vi "Word Report.vi"(6 "מק\"ט המכלל":string, 7 "עבר/נכשל":string="עבר/נכשל", 8 "מספר סידורי":string, 9 "שם הצב\"ד":string="שם הצב\"ד", 10 "מפעיל":string="ANS", 11 "Array":string[][](array[string])=[["Content", "Results", "Range", "Pass/Fail", "11"], ["Content", "Results", "Range", "Pass/Fail", "22"], ["Content", "Results", "Range", "Pass/Fail", "33"], ["Content", "Results", "Range", "Pass/Fail", "44"], ["Content", "Results", "Range", "Pass/Fail", "55"], ["55", "Content", "Results", "Range", "Pass/Fail"]]) -> ()   [LabVIEW 2014]
uses:
  <vilib>/addons/_office/_exclsub.llb/font.ctl
  <vilib>/addons/_office/word.llb/Word Easy Table (str).vi
  <vilib>/addons/_office/word.llb/Word Edit Cell ([str]).vi
  <vilib>/addons/_office/NI_ReportGenerationToolkit.lvlib
  <vilib>/Utility/NIReport.llb/Word/NI_Word.lvclass
panel:
  in  "start (0, 0)":cluster{"row":i32, "column":i32}={"row"=1, "column"=4}
  in  "value 3":string[][](array[string])
  in  "new element/subarray 3":string[](array[string])
  in  "new element/subarray":string[](array[string])
  in  "value":string[][](array[string])
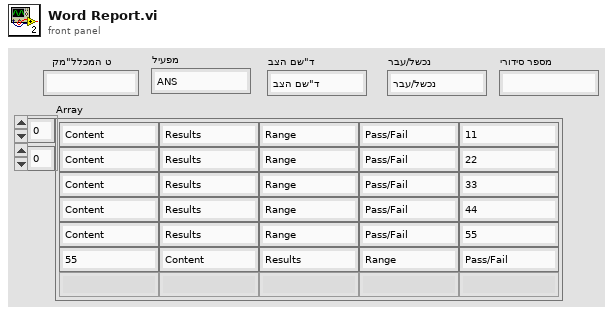
[diagram p1: front panel]
types:
  T1 = typedef "NI_ReportGenerationToolkit.lvlib/font.ctl" = cluster{"font name":string, "font size":dbl, "bold":u16, "italic":u16, "underline":u16, "strike through":u16, "font color":u32}
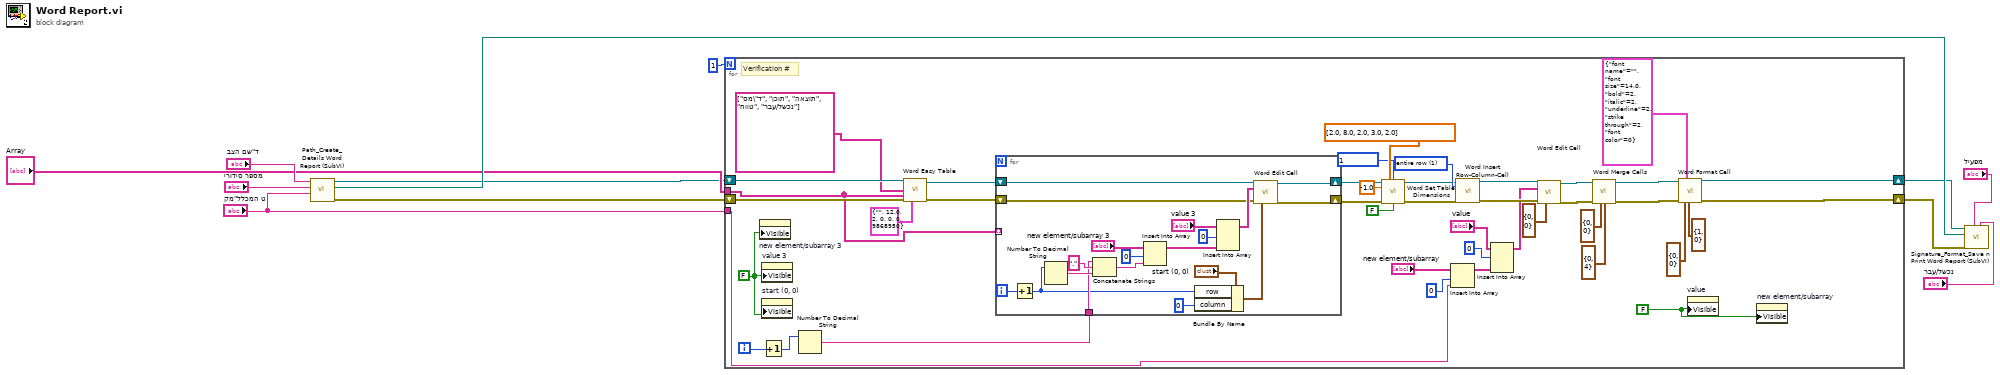
[diagram p0: block diagram]
diagram:
  n1 = call "Path_Create_Details Word Report (SubVI).vi"("שם ומק\"ט המכלל"="מק\"ט המכלל", "מספר סידורי"="מספר סידורי", "שם הצב\"ד"="שם הצב\"ד") -> ("error out"=w4:errorcluster, "Path"=w11:path, "NI_report out"=w5:refnum<class "NI_report.lvclass">)  [unwired: 6 in]
  n2 = for {
    N: 1 -> [_]
    shift-right: [w22] -> w9
    shift-left: w4 -> [w54]
    shift-right: [w23] -> w10
    shift-left: w5 -> [w53]
    tunnel: "Array" -> [w26]
    tunnel: "מק\"ט המכלל" -> [w14]
    i -> [w33]
    w34 = FALSE
    w40 = FALSE
    w52 = u16 1 items=["shift cells right", "entire row", "entire column"] ("mode (entire column)")
    # "Verification #"
    n3 = property on="new element/subarray 3" class="Arr (strict)"("Visible"=w34) -> ()  [unwired: 2 in, 2 out]
    n4 = property on="value 3" class="Arr (strict)"("Visible"=w34) -> ()  [unwired: 2 in, 2 out]
    n5 = property on="start (0, 0)" class="Clust (strict)"("Visible"=w34) -> ()  [unwired: 2 in, 2 out]
    n6 = Increment(x=w33) -> (x+1=w32:i32)
    n7 = Number To Decimal String(number=w32) -> (decimal integer string=w30:string)  [unwired: 1 in]
    n8 = call-poly <vilib>:"Word Easy Table.vi"("report in"=w53, "column headers"=string[] ["מס\"ד", "תוכן", "תוצאה", "טווח", "עבר/נכשל"], "data"=w26, "error in (no error)"=w54, "font"=T1 {"font name"="", "font size"=12.0, "bold"=2, "italic"=0, "underline"=0, "strike through"=0, "font color"=9868950}) -> ("report out"=w36:refnum<class "NI_report.lvclass">, "error out"=w35:errorcluster)  [unwired: 8 in, 1 out]
    n9 = for {
      shift-right: [w60] -> w21
      shift-left: w36 -> [w55]
      shift-right: [w59] -> w20
      shift-left: w35 -> [w56]
      tunnel: w30 -> [w64]
      tunnel: w26 -> [_] mode=indexing
      i -> [w61]
      n10 = Increment(x=w61) -> (x+1=w62:i32)
      n11 = Number To Decimal String(number=w62) -> (decimal integer string=w65:string)  [unwired: 1 in]
      n12 = Concatenate Strings(w64, ".", w65) -> (w67:string)
      n13 = Insert Into Array(array="new element/subarray 3", index=0, new element=w67) -> (w72:string[])
      n14 = Bundle By Name(cluster="start (0, 0)", "row"=w62, "column"=0) -> (w57:cluster{"row":i32, "column":i32})
      n15 = Insert Into Array(array="value 3", index (row)=0 ("disabled index (col)"), new element=w72) -> (w58:string[][])  [unwired: 1 in]
      n16 = call-poly <vilib>:"Word Edit Cell.vi"("report in"=w55, "value"=w58, "error in (no error)"=w56, "start (0, 0)"=w57) -> ("report out"=w60:refnum<class "NI_report.lvclass">, "error out"=w59:errorcluster)  [unwired: 10 in]
    }
    n17 = call <vilib>:"Word Set Table Dimensions.vi"("report in"=w21, "table column widths"=sgl[] [2.0, 8.0, 2.0, 3.0, 2.0], "measurement system"=u16 1, "left indent (0)"=sgl -1.0, "error in (no error)"=w20, "fit to page width? (F)"=FALSE) -> ("report out"=w18:refnum<class "NI_report.lvclass">, "error out"=w19:errorcluster)  [unwired: 8 in]
    n18 = Insert Into Array(array="new element/subarray", index=0, new element=w14) -> (w44:string[])
    n19 = call <vilib>:"Word Insert Row-Column-Cell.vi"("report in"=w18, "mode (entire column)"=w52, "error in (no error)"=w19) -> ("report out"=w51:refnum<class "NI_report.lvclass">, "error out"=w50:errorcluster)  [unwired: 11 in]
    n20 = Insert Into Array(array="value", index (row)=0, new element=w44) -> (w42:string[][])  [unwired: 1 in]
    n21 = call-poly <vilib>:"Word Edit Cell.vi"("report in"=w51, "value"=w42, "error in (no error)"=w50, "start (0, 0)"=cluster{"row":i32, "column":i32} {"row"=0, "column"=0}) -> ("report out"=w28:refnum<class "NI_report.lvclass">, "error out"=w27:errorcluster)  [unwired: 10 in]
    n22 = call <vilib>:"Word Merge Cells.vi"("report in"=w28, "error in (no error)"=w27, "start (0, 0)"=cluster{"start row":i32, "start column":i32} {"start row"=0, "start column"=0}, "end"=cluster{"end row":i32, "end column":i32} {"end row"=0, "end column"=4}) -> ("report out"=w25:refnum<class "NI_report.lvclass">, "error out"=w24:errorcluster)  [unwired: 10 in]
    n23 = call <vilib>:"Word Format Cell.vi"("report in"=w25, "font"=T1 {"font name"="", "font size"=14.0, "bold"=2, "italic"=2, "underline"=2, "strike through"=2, "font color"=0}, "error in (no error)"=w24, "start (-1, -1)"=cluster{"start row":i32, "start column":i32} {"start row"=1, "start column"=0}, "end (-1, -1)"=cluster{"end row":i32, "end column":i32} {"end row"=0, "end column"=0}) -> ("report out"=w23:refnum<class "NI_report.lvclass">, "error out"=w22:errorcluster)  [unwired: 9 in]
    n24 = property on="value" class="Arr (strict)"("Visible"=w40) -> ()  [unwired: 2 in, 2 out]
    n25 = property on="new element/subarray" class="Arr (strict)"("Visible"=w40) -> ()  [unwired: 2 in, 2 out]
  }
  n26 = call "Signature_Format_Save n Print Word Report (SubVI).vi"("עבר/נכשל"="עבר/נכשל", "מפעיל"="מפעיל", "error in (no error)"=w9, "Path"=w11, "NI_report in"=w10) -> ()  [unwired: 7 in]
